vi "Get Hardware Errors.vi"(8 "error in":errorcluster, 11 "Red-y Read Write CFG in":refnum<class "Red-y Pressure Control CFG.lvclass">) -> (0 "error out":errorcluster, 2 "Error Bits":T1, 3 "Red-y Read Write CFG out":refnum<class "Red-y Pressure Control CFG.lvclass">)   [LabVIEW 2023, in "Red-y Pressure Control CFG.lvclass"]
uses:
  Red-y Pressure Control CFG.lvclass
  Read Write PE Input.ctl
  <userlib>/_OpenG.lib/lvdata/lvdata.llb/Type Descriptor Enumeration__ogtk.ctl
  Red-y Pressure Control CFG.lvclass/Red-y Pressure Control CFG.ctl
  <userlib>/_OpenG.lib/lvdata/lvdata.llb/openg_variant.lvlib
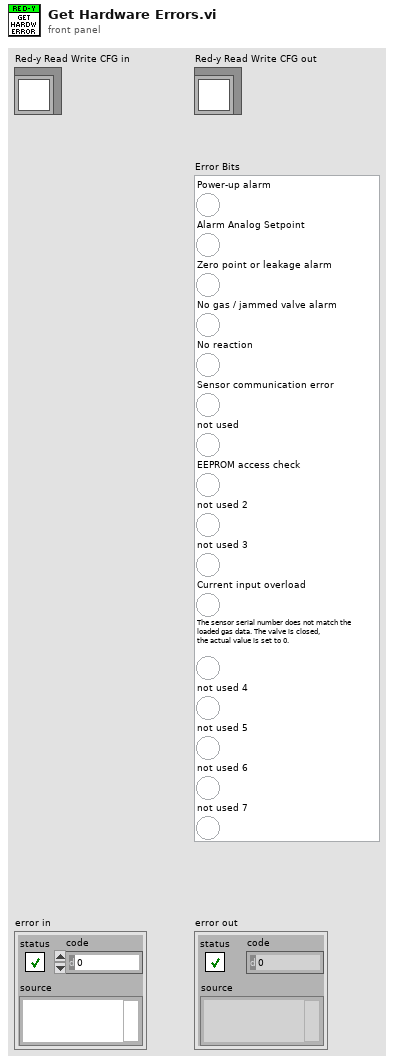
[diagram p1: front panel]
types:
  T1 = cluster{"Power-up alarm":bool, "Alarm Analog Setpoint":bool, "Zero point or leakage alarm":bool, "No gas / jammed valve alarm":bool, "No reaction":bool, "Sensor communication error":bool, "not used":bool, "EEPROM access check ":bool, "not used 2":bool, "not used 3":bool, "Current input overload":bool, "The sensor serial number does not match the \nloaded gas data. The valve is closed, \nthe actual value is set to 0.":bool, "not used 4":bool, "not used 5":bool, "not used 6":bool, "not used 7":bool}
  T2 = typedef "openg_variant.lvlib/Type Descriptor Enumeration__ogtk.ctl" = enum8{"<Null>", "I8", "I16", "I32", "I64", "U8", "U16", "U32", "U64", "SGL", "DBL", "EXT", "CSG", "CDB", "CXT", "0x0F", "0x10", "0x11", "0x12", "0x13", "0x14", "Enum U8", "Enum U16", "Enum U32", "Enum U64", "SGL PQ", "DBL PQ", "EXT PQ", "CSG PQ", "CDB PQ", "CXT PQ", "0x1F", "0x20", "Boolean", "0x22", "0x23", "0x24", "0x25", "0x26", "0x27", "0x28", "0x29", "0x2A", "0x2B", "0x2C", "0x2D", "0x2E", "0x2F", "String", "0x31", "Path", "Pict", "0x34", "0x35", "0x36", "DAQ", "0x38", "0x39", "0x3A", "0x3B", "0x3C", "0x3D", "0x3E", "0x3F", "Array", "0x41", "0x42", "0x43", "0x44", "0x45", "0x46", "0x47", "0x48", "0x49", "0x4A", "0x4B", "0x4C", "0x4D", "0x4E", "0x4F", "Cluster", "0x51", "0x52", "Variant", "Waveform", "0x55", "0x56", "0x57", "0x58", "0x59", "0x5A", "0x5B", "0x5C", "0x5D", "0x5E", "Fixed Point", "0x60", "0x61", "0x62", "0x63", "0x64", "0x65", "0x66", "0x67", "0x68", "0x69", "0x6A", "0x6B", "0x6C", "0x6D", "0x6E", "0x6F", "Refnum", "0x71", "0x72", "Set Collection", "Map Collection"}
  T3 = typedef "Read Write PE Input.ctl" = cluster{"Action":enum16{"Write", "Read"}, "Register":u16, "Type":T2, "Data":variant}
  T4 = cluster{"Boolean array[0]":bool, "Boolean array[1]":bool, "Boolean array[2]":bool, "Boolean array[3]":bool, "Boolean array[4]":bool, "Boolean array[5]":bool, "Boolean array[6]":bool, "Boolean array[7]":bool, "Boolean array[8]":bool, "Boolean array[9]":bool, "Boolean array[10]":bool, "Boolean array[11]":bool, "Boolean array[12]":bool, "Boolean array[13]":bool, "Boolean array[14]":bool, "Boolean array[15]":bool}
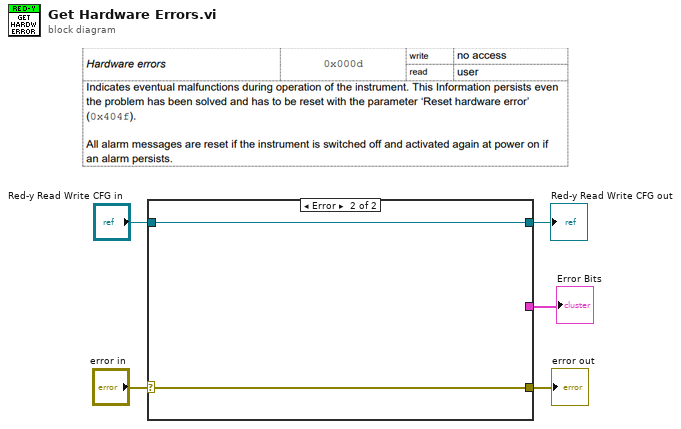
[diagram p0: block diagram]
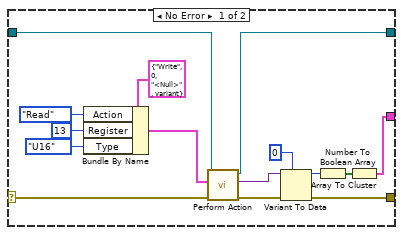
[diagram p2: hidden frame]
diagram:
  n1 = case shown="Error" "error in" {
    selector: "error in" -> [w13 w22]
    tunnel: [w11 w22] -> w4
    tunnel: [w14 w21] -> w2
    tunnel: "Red-y Read Write CFG in" -> [w15 w21]
    tunnel: [w8 _] -> w1
    frame No Error {
      n2 = Bundle By Name(cluster=T3 {"Action"=enum."Write", "Register"=0, "Type"=enum."<Null>", "Data"=variant}, "Action"=enum16{"Write", "Read"}."Read", "Register"=u16 13 ("Register Start Address"), "Type"=Type_Descriptor_Enumeration__ogtk."U16") -> (w19:T3)
      n3 = call-dynamic "Perform Action.vi"("error in"=w13, "Input"=w19, "Red-y Read Write CFG in"=w15) -> ("error out"=w12:errorcluster, "Output"=w10:variant, "Red-y Read Write CFG out"=w14:refnum<class "Red-y Pressure Control CFG.lvclass">)  [unwired: 6 in]
      n4 = Variant To Data(error in=w12, type=u16 0, Variant=w10) -> (data=w6:u16, error out=w11:errorcluster)
      n5 = Number To Boolean Array(number=w6) -> (Boolean array=w9:bool[])
      n6 = Array To Cluster(array=w9) -> (cluster=w8:T4)
    }
    frame Error {
    }
  }
  "error out" <- w4
  "Red-y Read Write CFG out" <- w2
  "Error Bits" <- w1
